vi "Generate Configuration Error.vi"(8 "error in (no error)":errorcluster, 10 "JSON":string, 11 "Key":string) -> (0 "error out":errorcluster)   [LabVIEW 2020, in "Error Provider API.lvlib"]
uses:
  <vilib>/NI VeriStand/Error Provider API/Error Provider API.lvlib
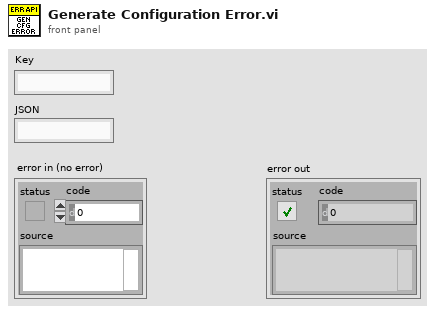
[diagram p1: front panel]
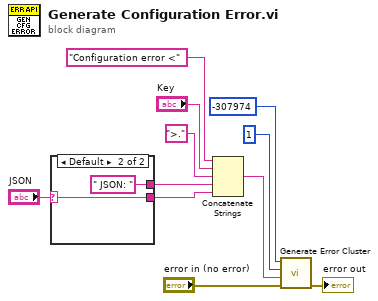
[diagram p0: block diagram]
diagram:
  n1 = case shown="Default" "JSON" {
    selector: "JSON" -> [_ w12]
    tunnel: [_ " JSON: " ("string")] -> w8
    tunnel: [_ w12] -> w2
    frame "" {
    }
    frame Default {
    }
  }
  n2 = Concatenate Strings("Configuration error <" ("Additional Message"), "Key", ">." ("string"), w8, w2) -> (w9:string)
  n3 = call <vilib>:"Generate Error Cluster.vi"("error in (no error)"="error in (no error)", "Additional Message"=w9, "CallChainLvl (-1 => No call chain)"=1, "Code"=-307974) -> ("error out"=→"error out":errorcluster)  [unwired: 7 in]
